vi "ExReadPMIFile.vi"() -> ()   [LabVIEW 2010]
panel:
  in  "Full File Name":path
  in  "?":bool
  out "error out":errorcluster
  in  "error in (no error)":errorcluster
  # "ExReadPMIFile.vi\nThis VI will read a PMI type image file and\ndisplay it.  Be sure to hit the CLOSE IMAGE\nbutton when finished viewing the image so\nit is closed and memory is deallocated\nproperly"
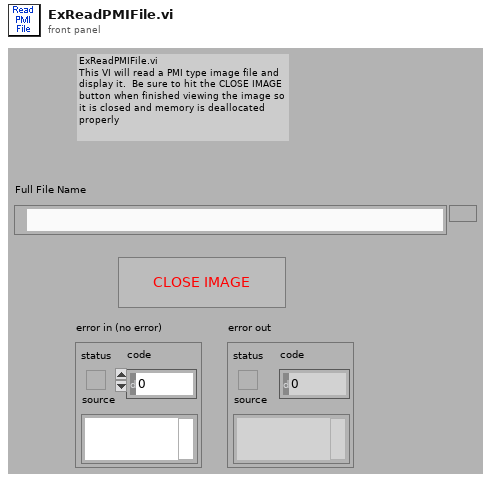
[diagram p1: front panel]
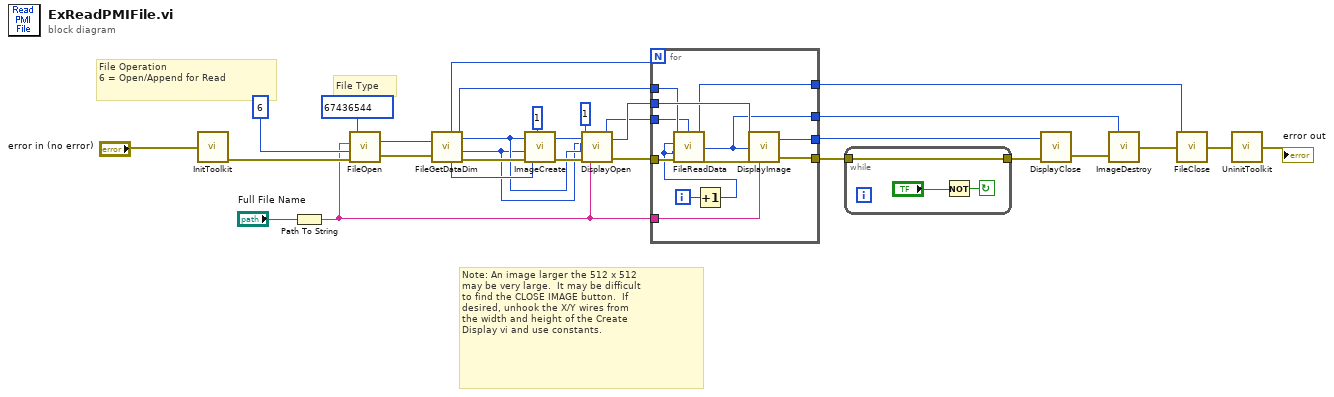
[diagram p0: block diagram]
diagram:
  # "File Type"
  # "File Operation\n6 = Open/Append for Read"
  # "Note: An image larger the 512 x 512\nmay be very large.  It may be difficult\nto find the CLOSE IMAGE button.  If\ndesired, unhook the X/Y wires from\nthe width and height of the Create\nDisplay vi and use constants."
  n1 = call <userlib>:"InitToolkit.vi"("error in"="error in (no error)") -> ("error out"=w27:errorcluster)
  n2 = Path To String(path="Full File Name") -> (string=w3:string)
  n3 = call <userlib>:"FileOpen.vi"("error in"=w27, "File Operations"=u32 6 ("File Operation"), "FileName"=w3, "File Type"=u32 67436544 ("FileType")) -> ("error out"=w25:errorcluster, "File Handle"=w24:u32)
  n4 = call <userlib>:"FileGetDataDim.vi"("File Handle"=w24, "error in"=w25) -> ("Number of Frames"=w20:u32, "Data Type"=w22:u32, "File Handle"=w15:u32, "X dim"=w2:u32, "Y dim"=w1:u32, "error out"=w23:errorcluster)
  n5 = call <userlib>:"ImageCreate.vi"("X dimension"=w2, "Y dimension"=w1, "Data Type"=w22, "error in"=w23, "Number Of Frames"=1) -> ("Image Handle"=w14:u32, "error out"=w21:errorcluster)
  n6 = call <userlib>:"DisplayOpen.vi"("Display Title"=w3, "Image Handle"=w14, "error in"=w21, "Display Height"=w1, "Display Width"=w2, "Display Type"=1) -> ("error out"=w17:errorcluster, "Display Handle"=w16:u32)
  n7 = for {
    N: w20 -> [_]
    tunnel: w17 -> [w41]
    tunnel: w16 -> [w39]
    tunnel: w15 -> [w38]
    tunnel: w14 -> [w37]
    tunnel: [w34] -> w5
    tunnel: [w33] -> w13
    tunnel: [w32] -> w12
    tunnel: [w31] -> w9
    tunnel: w3 -> [w30]
    i -> [w36]
    n8 = Increment(x=w36) -> (x+1=w35:i32)
    n9 = call <userlib>:"FileReadData.vi"("File Handle"=w38, "Start Frame"=w35, "End Frame"=w35, "error in"=w41, "Image Handle"=w37) -> ("File Handle"=w32:u32, "Image Handle"=w31:u32, "error out"=w40:errorcluster)
    n10 = call <userlib>:"DisplayImage.vi"("error in"=w40, "Title"=w30, "Image Handle"=w31, "Display Handle"=w39) -> ("error out"=w34:errorcluster, "Display Handle"=w33:u32)
  }
  n11 = while {
    tunnel: w5 -> [w44]
    tunnel: [w44] -> w6
    stop <- w42 continue-if-true
    n12 = Not(x="?") -> (.not. x?=w42:bool)
  }
  n13 = call <userlib>:"DisplayClose.vi"("error in"=w6, "Display Handle"=w13) -> ("error out"=w11:errorcluster)
  n14 = call <userlib>:"ImageDestroy.vi"("error in"=w11, "Data handle"=w9) -> ("error out"=w10:errorcluster)
  n15 = call <userlib>:"FileClose.vi"("error in"=w10, "File Handle"=w12) -> ("error out"=w8:errorcluster)
  n16 = call <userlib>:"UninitToolkit.vi"("error in"=w8) -> ("error out"=→"error out":errorcluster)
